vi "FTW-Scripter-Test.vi"() -> ()   [LabVIEW 2015]
uses:
  templates/Scripter Steps/Wait/core/FTW-ScripterStep-Wait-Core_Step.vi
  source/actor/Connector/FTW-ActorConnector.lvclass
  templates/Scripter Steps/Wait/core/FTW-ScripterStep-Wait-Core.lvclass
panel:
  in  "Start":bool
  in  "Load":bool
  out "Multicolumn Listbox":i32(listbox)
  out "error out":errorcluster
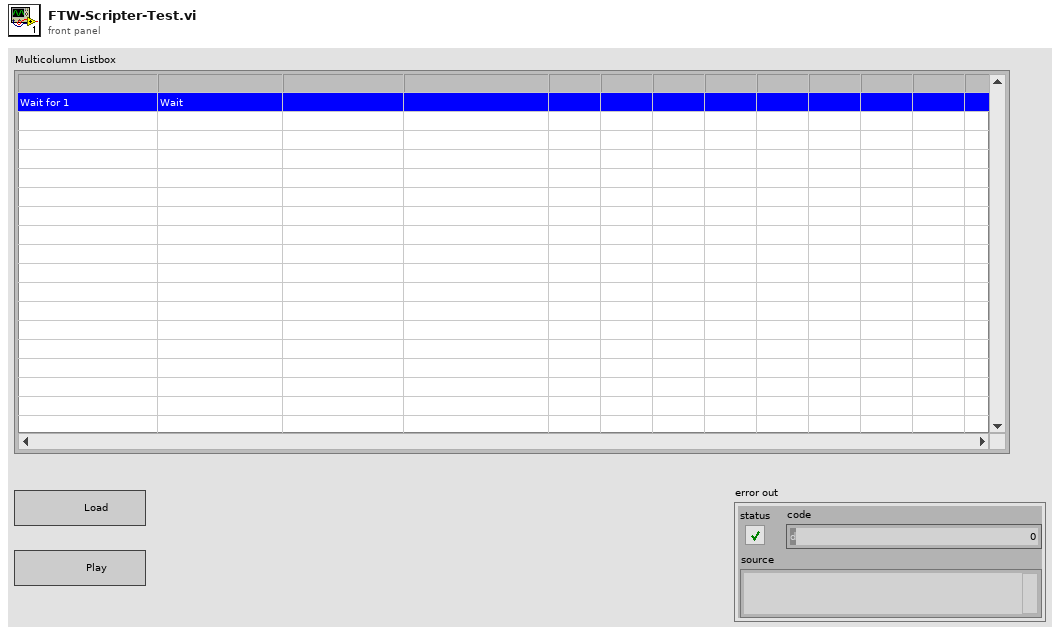
[diagram p1: front panel]
types:
  T1 = typedef "FTW-Scripter_Step.ctl" = cluster{"Name":string, "Type":string, "Path":string, "Config":string}
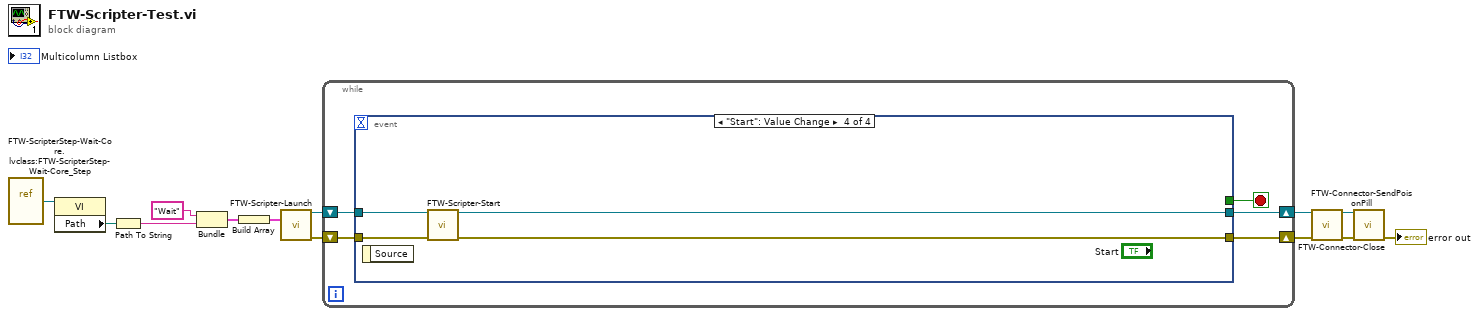
[diagram p0: block diagram]
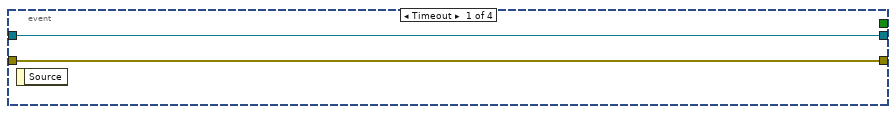
[diagram p2: hidden frame]
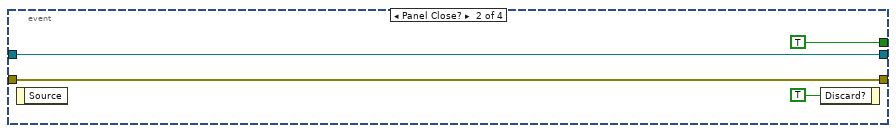
[diagram p3: hidden frame]
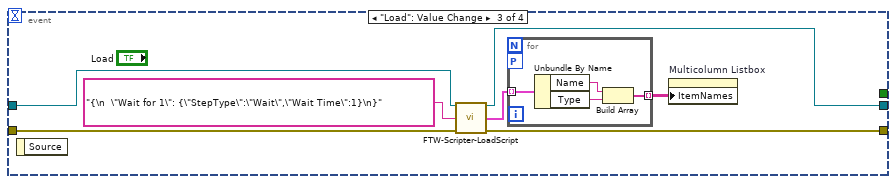
[diagram p4: hidden frame]
diagram:
  n1 = vi-ref "FTW-ScripterStep-Wait-Core.lvclass:FTW-ScripterStep-Wait-Core_Step.vi"() -> (w10:refnum<vi>)
  n2 = property class="VI"(reference=w10) -> ("Path"=w8:path)  [unwired: 1 in, 2 out]
  n3 = Path To String(path=w8) -> (string=w7:string)
  n4 = Bundle("Wait", w7) -> (w6:cluster{string, string})  [unwired: 1 in]
  n5 = Build Array(w6) -> (w5:cluster{string, string}[])
  n6 = call "FTW-Scripter-Launch.vi"("Step Name Dictionary"=w5) -> ("FTW Actor Connector"=w4:refnum<class "FTW-ActorConnector.lvclass">, "error out"=w3:errorcluster)  [unwired: 11 in, 2 out]
  n7 = while {
    shift-right: [w14] -> w1
    shift-left: w4 -> [w17]
    shift-right: [w15] -> w2
    shift-left: w3 -> [w16]
    stop <- w18 stop-if-true
    n8 = event shown="[3] \"Start\": Value Change" {
      selector: _ -> [_ _ _ _]
      dyn-events: _ -> [_ _ _ _]
      timeout: _ -> [_ _ _ _]
      tunnel: [_ TRUE _ _] -> w18
      tunnel: w17 -> [w19 w23 w31 w37]
      tunnel: w16 -> [w20 w24 w30 w39]
      tunnel: [w20 w24 w29 w38] -> w15
      tunnel: [w19 w23 w28 w36] -> w14
      event Timeout {
        n9 = event-data() -> ()  [unwired: 1 in, 1 out]
      }
      event Panel Close? {
        n10 = event-data() -> ()  [unwired: 1 in, 1 out]
        n11 = event-data("Discard?"=TRUE) -> ()  [unwired: 1 in, 1 out]
      }
      event "Load": Value Change {
        n12 = event-data() -> ()  [unwired: 1 in, 1 out]
        n13 = call "FTW-Scripter-LoadScript.vi"("FTW Actor Connector In"=w31, "Script"="{\n  \"Wait for 1\": {\"StepType\":\"Wait\",\"Wait Time\":1}\n}", "error in (no error)"=w30) -> ("FTW Actor Connector"=w28:refnum<class "FTW-ActorConnector.lvclass">, "Loaded Script"=w26:T1[], "error out"=w29:errorcluster)  [unwired: 9 in, 1 out]
        n14 = for {
          tunnel: w26 -> [w35] mode=indexing
          tunnel: [w32] -> w25 mode=indexing
          workers-P: _ -> [_]
          n15 = Unbundle By Name(w35) -> ("Name"=w34:string, "Type"=w33:string)
          n16 = Build Array(w34, w33) -> (w32:string[])
        }
        n17 = property on="Multicolumn Listbox" class="MCListbox (strict)"("ItemNames"=w25) -> ()  [unwired: 2 in, 2 out]
      }
      event "Start": Value Change {
        n18 = event-data() -> ()  [unwired: 1 in, 1 out]
        n19 = call "FTW-Scripter-Start.vi"("FTW Actor Connector In"=w37, "error in (no error)"=w39) -> ("FTW Actor Connector"=w36:refnum<class "FTW-ActorConnector.lvclass">, "error out"=w38:errorcluster)  [unwired: 10 in, 2 out]
      }
    }
  }
  n20 = call-dynamic "FTW-Connector-SendPoisonPill.vi"("FTW Actor Connector"=w1, "error in"=w2) -> ("FTW Actor Connector out"=w11:refnum<class "FTW-ActorConnector.lvclass">, "error out"=w12:errorcluster)  [unwired: 8 in, 4 out]
  n21 = call-dynamic "FTW-Connector-Close.vi"("FTW Actor Connector"=w11, "error in"=w12) -> ("error out"=→"error out":errorcluster)  [unwired: 13 in]
